vi "TransComm_ReadFilePackets.vi"(8 "error in (no error)":errorcluster, 10 "chunk size":i32, 11 "File Ref":refnum<file>) -> (0 "error out":errorcluster, 1 "EOF":bool=TRUE, 2 "Data":u8[](array[numeric]), 3 "File Ref out":refnum<file>)   [LabVIEW 2017, in "ServerComm.lvlib"]
uses:
  <vilib>/addons/InsightCM/Devices/Shared/Common/ServerComm/ServerComm.lvlib
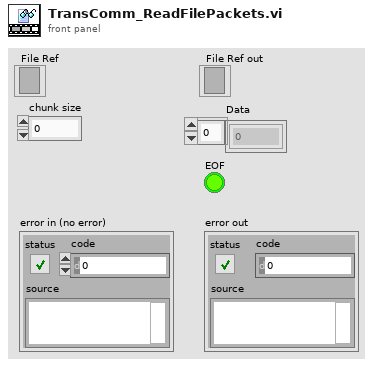
[diagram p1: front panel]
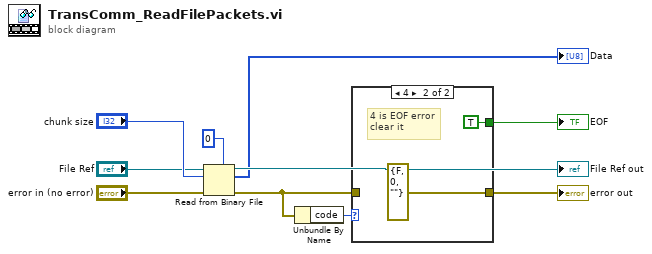
[diagram p0: block diagram]
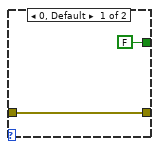
[diagram p2: hidden frame]
diagram:
  n1 = Read from Binary File(5:u8 0, 8:"error in (no error)", 10:"chunk size", 11:"File Ref") -> (0:w9:errorcluster, 2:→"Data":u8[], 3:→"File Ref out":refnum<file>)  [unwired: 2 in, 1 out]
  n2 = Unbundle By Name(w9) -> ("code"=w8:i32)
  n3 = case shown="4" w8 {
    tunnel: w9 -> [w12 _]
    tunnel: [w12 errorcluster {"status"=FALSE, "code"=0, "source"=""} ("error out")] -> w10
    tunnel: [FALSE TRUE] -> w2
    frame 0, Default {
    }
    frame 4 {
      # "4 is EOF error\nclear it"
    }
  }
  "EOF" <- w2
  "error out" <- w10
